vi "has_GUI.vi"(8 "error in (no error)":errorcluster, 11 "DL090628DSSTraceProcessor in":refnum<class "TraceProcessorDL091210Raw.lvclass">) -> (0 "error out":errorcluster, 2 "has GUI?":bool, 3 "DL090628DSSTraceProcessor out":refnum<class "TraceProcessorDL091210Raw.lvclass">)   [LabVIEW 2010, in "TraceProcessorDL091210Raw.lvclass"]
uses:
  TraceProcessorDL091210Raw.lvclass
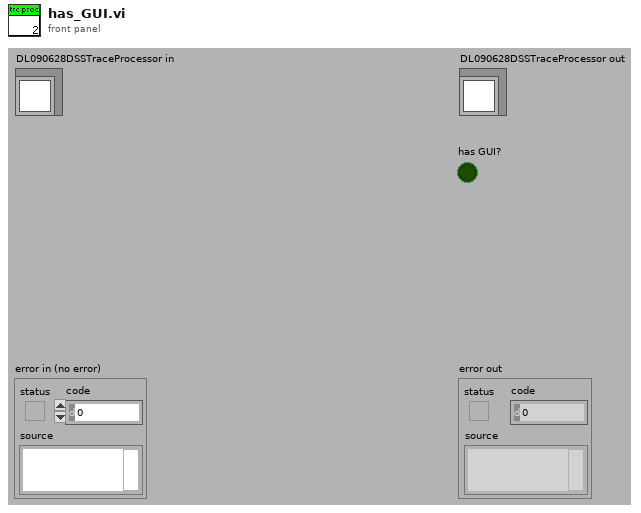
[diagram p1: front panel]
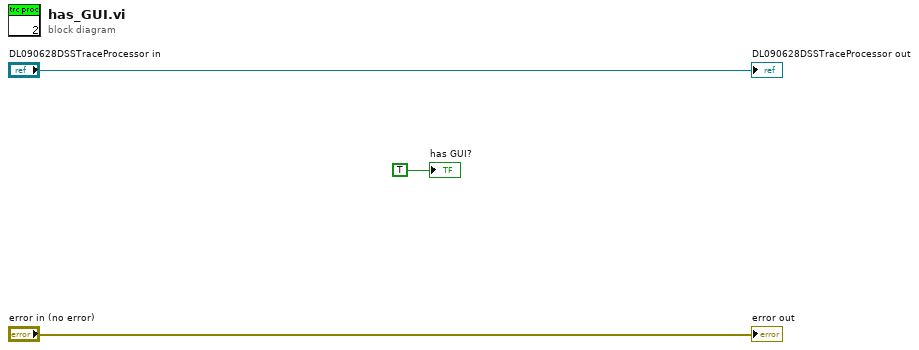
[diagram p0: block diagram]
diagram:
  "error out" <- "error in (no error)"
  "DL090628DSSTraceProcessor out" <- "DL090628DSSTraceProcessor in"
  "has GUI?" <- TRUE
